vi "Week 3 Practical - Prof Base.vi"() -> ()   [LabVIEW 2013]
panel:
  in  "stop":bool
  in  "Operation":string(combo)="Select Op"
  in  "Operand X":dbl
  in  "Operand Y":dbl
  out "1SQ RES":dbl
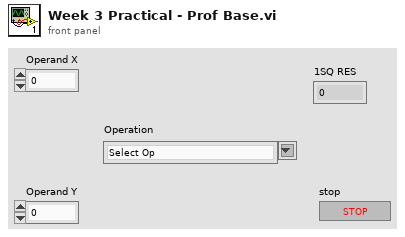
[diagram p1: front panel]
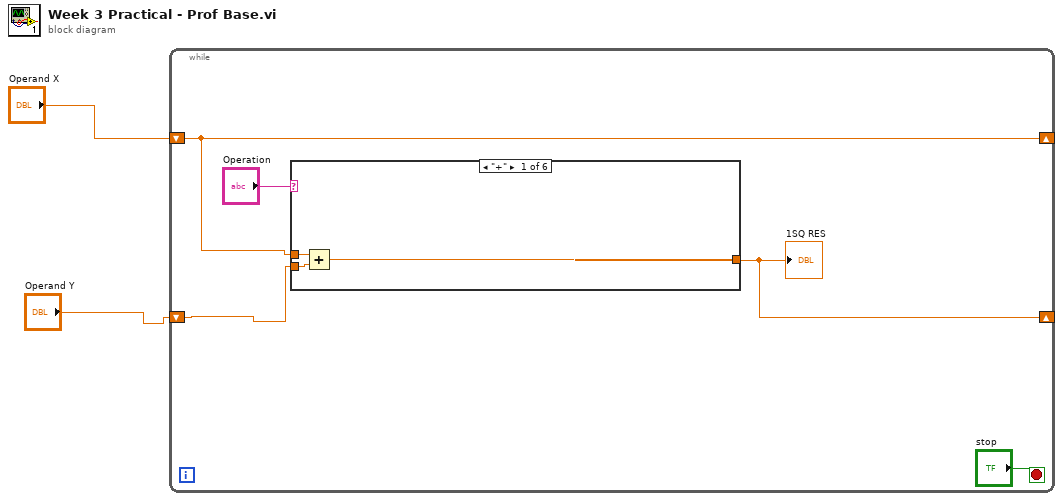
[diagram p0: block diagram]
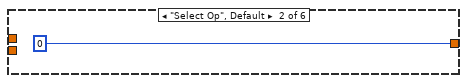
[diagram p2: hidden frame]
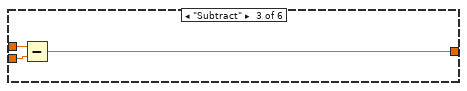
[diagram p3: hidden frame]
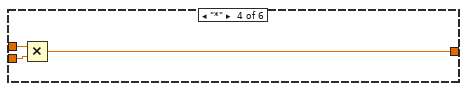
[diagram p4: hidden frame]
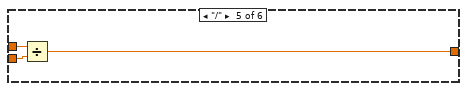
[diagram p5: hidden frame]
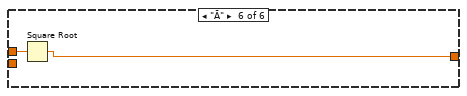
[diagram p6: hidden frame]
diagram:
  n1 = while {
    shift-right: [w3] -> _
    shift-left: "Operand X" -> [w3]
    shift-right: [w4] -> _
    shift-left: "Operand Y" -> [w5]
    stop <- "stop" stop-if-true
    n2 = case shown="\"+\"" "Operation" {
      tunnel: w5 -> [w9 _ w13 w16 w19 _]
      tunnel: w3 -> [w10 _ w14 w17 w20 w22]
      tunnel: [w8 0 w12 w15 w18 w21] -> w4
      frame "+" {
        n3 = Add(x=w10, y=w9) -> (x+y=w8:dbl)
      }
      frame "Select Op", Default {
      }
      frame "Subtract" {
        n4 = Subtract(x=w14, y=w13) -> (x-y=w12:dbl)
      }
      frame "*" {
        n5 = Multiply(x=w17, y=w16) -> (x*y=w15:dbl)
      }
      frame "/" {
        n6 = Divide(x=w20, y=w19) -> (x/y=w18:dbl)
      }
      frame "Ã" {
        n7 = Square Root(x=w22) -> (sqrt(x)=w21:dbl)
      }
    }
    "1SQ RES" <- w4
  }
